vi "MultiTool-Track-Generate-ndipolarisFileOutput-Q-vectors-Accepts Joystick Command with Time Display-Testing tcp time stamp.vi"() -> ()   [LabVIEW 2013]
panel:
  out "TIME":string
  out "bytes written":i32
  out "Return time string":string
  out "Length":u8
  out "Command":u8
  out "Tool 2":T1={"Port Handle"="", "Frame Number"=0, "Tx"=0.0, "Ty"=0.0, "Tz"=0.0, "Q0"=0.0, "Qx"=0.0, "Qy"=0.0, "Qz"=0.0, "Deviation"=0.0, " Markers Missing"=TRUE, "Out of Volume"=TRUE} {"Deviation" format="%#.4f"; "Qz" format="%#.4f"; "Qy" format="%#.4f"; "Qx" format="%#.4f"; "Q0" format="%#.4f"; "Tz" format="%#.2f"; "Ty" format="%#.2f"; "Tx" format="%#.2f"}
  in  "Location of ROM File for Tool 2":path=path "C:/Program Files (x86)/Northern Digital Inc/8700339.rom"
  in  "NDI  Running":bool=TRUE
  out "Stop Reading":bool=TRUE
  out "Start Reading":bool
  out "Object Identifier":string="0"
  in  "Track Outside Measurement Volume? (F:No)":bool
  in  "Track Stray Markers? (F:No)":bool
  out "Tool 1":T1={"Port Handle"="", "Frame Number"=0, "Tx"=0.0, "Ty"=0.0, "Tz"=0.0, "Q0"=0.0, "Qx"=0.0, "Qy"=0.0, "Qz"=0.0, "Deviation"=0.0, " Markers Missing"=TRUE, "Out of Volume"=TRUE} {"Deviation" format="%#.4f"; "Qz" format="%#.4f"; "Qy" format="%#.4f"; "Qx" format="%#.4f"; "Q0" format="%#.4f"; "Tz" format="%#.2f"; "Ty" format="%#.2f"; "Tx" format="%#.2f"}
  out "TCP loop":i32
  in  "TCP Server Running":bool=TRUE
  in  "Output Directory":path=path "C:/Users/Diogo/Desktop/NDI-Labview Gripper"
  out "NDI Loop":i32
  in  "VISA resource name":refnum<visa-resource-name>="COM8"
  in  "Reset? (T:Yes)":bool=TRUE
  in  "Location of ROM File for Tool 1":path=path "C:/Program Files (x86)/Northern Digital Inc/8700449.rom"
  in  "Serial Configuration":T2={"Baud Rate (9600)"=9600, "Flow Control (0:None)"=0, "Parity"=0, "Data Bits"=8, "Stop Bits"=10} {"Stop Bits" items=["1.0"=10, "2.0"=20]; "Parity" items=["None", "Odd", "Even"]; "Flow Control (0:None)" items=["None", "XON/XOFF"]; "Baud Rate (9600)" items=["9600"=9600, "14.4k"=14400, "19.2k"=19200, "38.4k"=38400, "57.6k "=57600, "115.2k"=115200]}
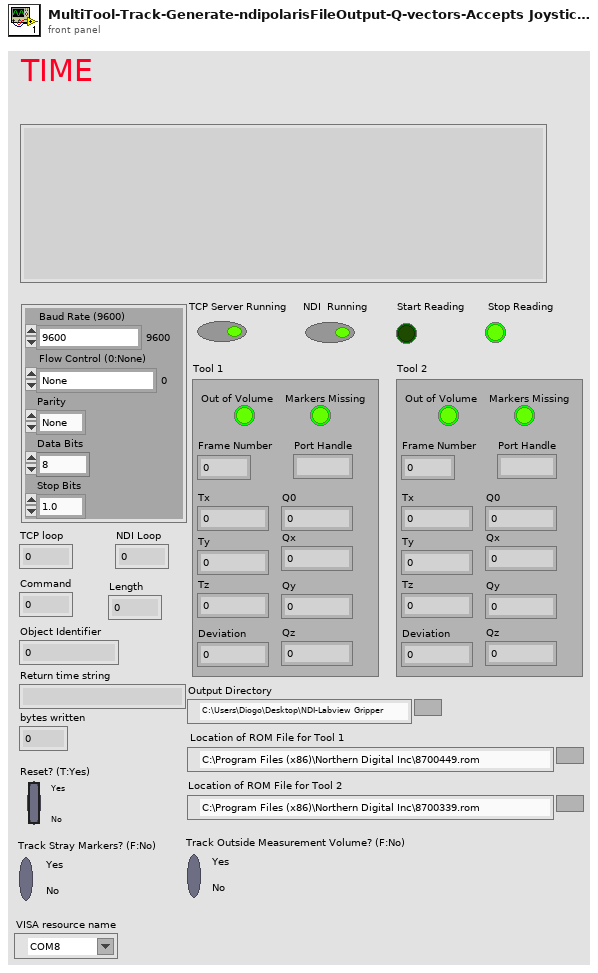
[diagram p1: front panel]
types:
  T1 = cluster{"Port Handle":string, "Frame Number":i32, "Tx":dbl, "Ty":dbl, "Tz":dbl, "Q0":dbl, "Qx":dbl, "Qy":dbl, "Qz":dbl, "Deviation":dbl, " Markers Missing":bool, "Out of Volume":bool}
  T2 = cluster{"Baud Rate (9600)":u32, "Flow Control (0:None)":u16, "Parity":u16, "Data Bits":u16, "Stop Bits":u16}
  T3 = cluster{"Port Handle":string, "Frame Number":u32, "Tx":dbl, "Ty":dbl, "Tz":dbl, "Q0":dbl, "Qx":dbl, "Qy":dbl, "Qz":dbl, "Deviation":dbl, "Missing?":bool, "Out of Volume?":bool}[]
  T4 = cluster{"Transformations[0]":cluster{"Port Handle":string, "Frame Number":u32, "Tx":dbl, "Ty":dbl, "Tz":dbl, "Q0":dbl, "Qx":dbl, "Qy":dbl, "Qz":dbl, "Deviation":dbl, "Missing?":bool, "Out of Volume?":bool}, "Transformations[1]":cluster{"Port Handle":string, "Frame Number":u32, "Tx":dbl, "Ty":dbl, "Tz":dbl, "Q0":dbl, "Qx":dbl, "Qy":dbl, "Qz":dbl, "Deviation":dbl, "Missing?":bool, "Out of Volume?":bool}, "Transformations[2]":cluster{"Port Handle":string, "Frame Number":u32, "Tx":dbl, "Ty":dbl, "Tz":dbl, "Q0":dbl, "Qx":dbl, "Qy":dbl, "Qz":dbl, "Deviation":dbl, "Missing?":bool, "Out of Volume?":bool}, "Transformations[3]":cluster{"Port Handle":string, "Frame Number":u32, "Tx":dbl, "Ty":dbl, "Tz":dbl, "Q0":dbl, "Qx":dbl, "Qy":dbl, "Qz":dbl, "Deviation":dbl, "Missing?":bool, "Out of Volume?":bool}, "Transformations[4]":cluster{"Port Handle":string, "Frame Number":u32, "Tx":dbl, "Ty":dbl, "Tz":dbl, "Q0":dbl, "Qx":dbl, "Qy":dbl, "Qz":dbl, "Deviation":dbl, "Missing?":bool, "Out of Volume?":bool}, "Transformations[5]":cluster{"Port Handle":string, "Frame Number":u32, "Tx":dbl, "Ty":dbl, "Tz":dbl, "Q0":dbl, "Qx":dbl, "Qy":dbl, "Qz":dbl, "Deviation":dbl, "Missing?":bool, "Out of Volume?":bool}, "Transformations[6]":cluster{"Port Handle":string, "Frame Number":u32, "Tx":dbl, "Ty":dbl, "Tz":dbl, "Q0":dbl, "Qx":dbl, "Qy":dbl, "Qz":dbl, "Deviation":dbl, "Missing?":bool, "Out of Volume?":bool}, "Transformations[7]":cluster{"Port Handle":string, "Frame Number":u32, "Tx":dbl, "Ty":dbl, "Tz":dbl, "Q0":dbl, "Qx":dbl, "Qy":dbl, "Qz":dbl, "Deviation":dbl, "Missing?":bool, "Out of Volume?":bool}, "Transformations[8]":cluster{"Port Handle":string, "Frame Number":u32, "Tx":dbl, "Ty":dbl, "Tz":dbl, "Q0":dbl, "Qx":dbl, "Qy":dbl, "Qz":dbl, "Deviation":dbl, "Missing?":bool, "Out of Volume?":bool}}
  T5 = cluster{"Port Handle":string, "Frame Number":u32, "Tx":dbl, "Ty":dbl, "Tz":dbl, "Q0":dbl, "Qx":dbl, "Qy":dbl, "Qz":dbl, "Deviation":dbl, "Missing?":bool, "Out of Volume?":bool}
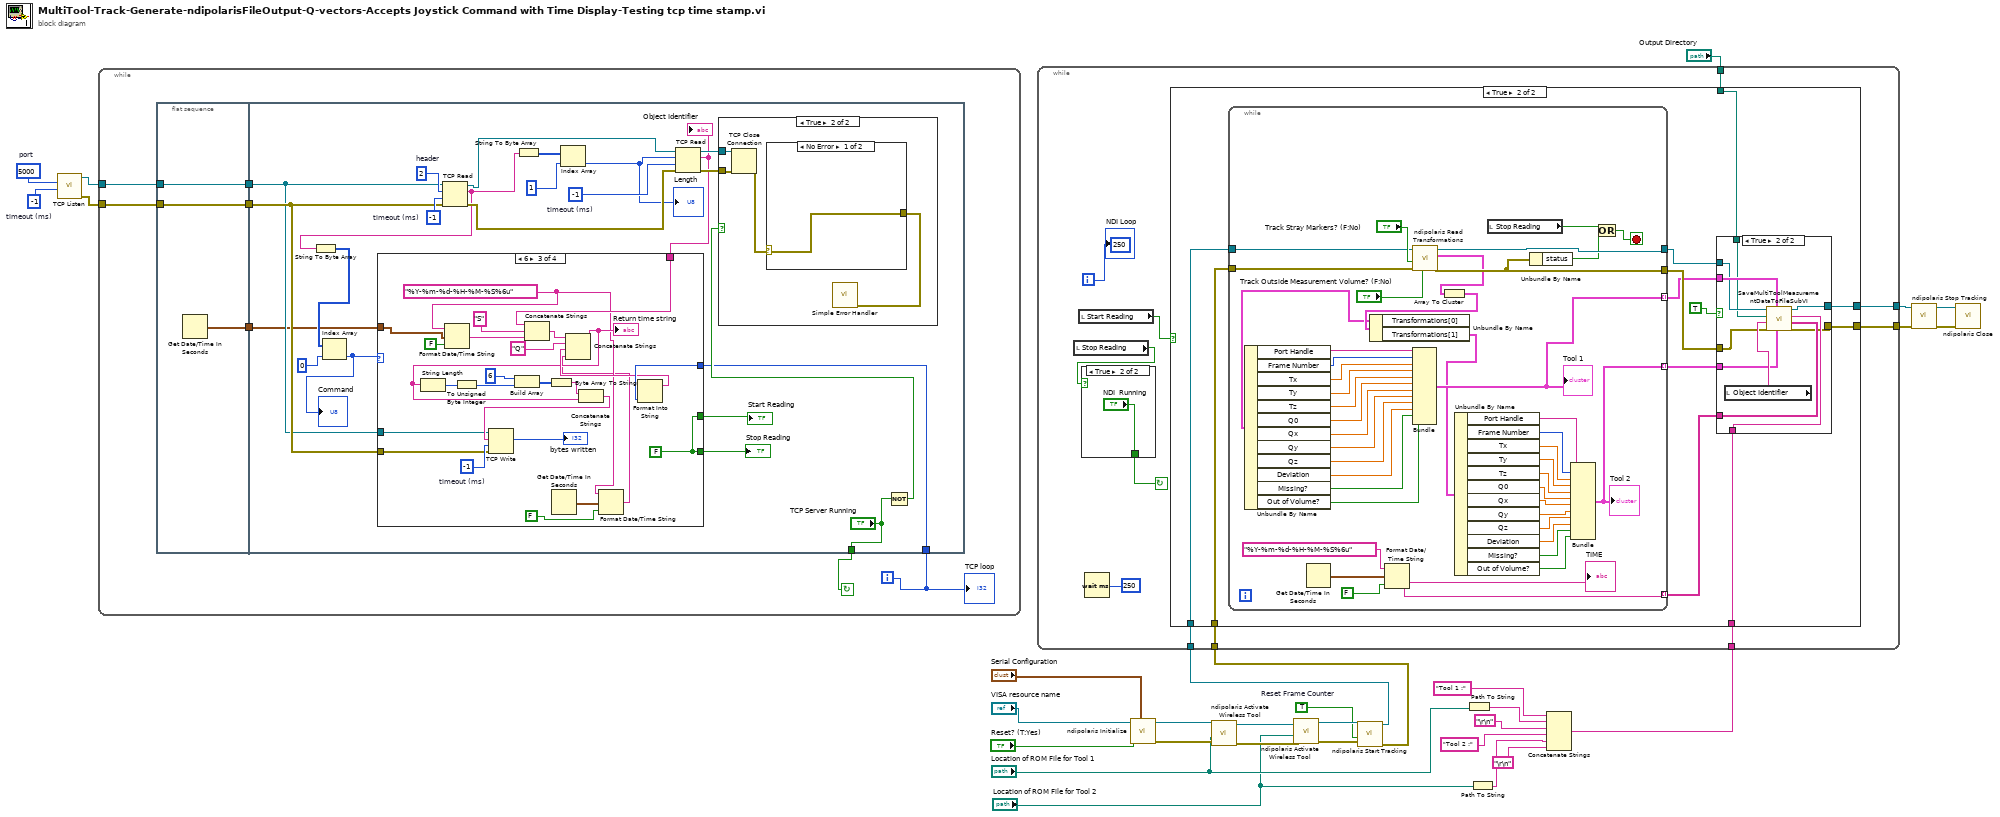
[diagram p0: block diagram]
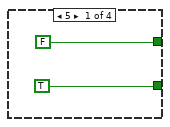
[diagram p2: hidden frame]
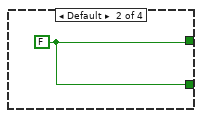
[diagram p3: hidden frame]
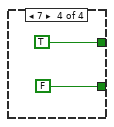
[diagram p4: hidden frame]
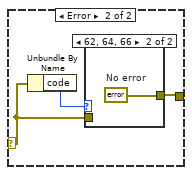
[diagram p6: hidden frame]
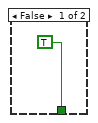
[diagram p8: hidden frame]
diagram:
  w21 = TRUE  # Reset Frame Counter
  w30 = u16 5000  # port
  w29 = i8 -1  # timeout (ms)
  n1 = call <vilib>:"TCP Listen.vi"("timeout ms (wait forever: -1)"=w29, "port"=w30) -> ("error out"=w24:errorcluster, "connection ID"=w25:refnum<k5>)  [unwired: 5 in, 3 out]
  n2 = while {
    tunnel: w25 -> [w35]
    tunnel: w24 -> [w36]
    i -> [w31]
    stop <- w37 continue-if-true
    n3 = flat-sequence {
      tunnel: w35 -> [w39]
      tunnel: w36 -> [w40]
      tunnel: [w40] -> w34
      tunnel: [w39] -> w33
      tunnel: [w38] -> w32
      tunnel: ["TCP Server Running"] -> w37
      tunnel: w34 -> [w45]
      tunnel: w33 -> [w43]
      tunnel: w32 -> [w42]
      tunnel: w31 -> [w41]
      frame #0 {
        n4 = Get Date/Time In Seconds() -> (seconds since 1Jan1904=w38:timestamp)
      }
      frame #1 {
        w59 = i8 -1  # timeout (ms)
        w62 = i8 -1  # timeout (ms)
        w63 = i8 2  # header
        n5 = TCP Read(connection ID=w43, bytes to read=w63, error in (no error)=w45, 9:w62) -> (connection ID out=w61:refnum<k5>, data out=w50:string, error out=w60:errorcluster)  [unwired: 1 in]
        n6 = String To Byte Array(string=w50) -> (unsigned byte array=w53:u8[])
        n7 = Index Array(array=w53, index=0) -> (element=w46:u8)
        "Command" <- w46
        n8 = String To Byte Array(string=w50) -> (unsigned byte array=w52:u8[])
        n9 = Index Array(array=w52, index=1) -> (element=w49:u8)
        "Length" <- w49
        n10 = TCP Read(connection ID=w61, bytes to read=w49, error in (no error)=w60, 9:w59) -> (connection ID out=w58:refnum<k5>, data out=w44:string, error out=w57:errorcluster)  [unwired: 1 in]
        "Object Identifier" <- w44
        n11 = case shown="6" w46 {
          tunnel: [FALSE w66 w77 TRUE] -> w56
          tunnel: [TRUE w66 w77 FALSE] -> w55
          tunnel: w45 -> [_ _ w80 _]
          tunnel: w44 -> [_ _ w79 _]
          tunnel: w43 -> [_ _ w78 _]
          tunnel: w42 -> [_ _ w76 _]
          tunnel: w41 -> [_ _ w73 _]
          frame 5 {
          }
          frame Default {
            w66 = FALSE
          }
          frame 6 {
            w88 = i8 -1  # timeout (ms)
            w68 = "%Y-%m-%d-%H-%M-%S%6u"
            w77 = FALSE
            n12 = Format Date/Time String(time format string (%c)=w68, seconds (now)=w76, UTC format=FALSE) -> (date/time string=w91:string)
            n13 = Concatenate Strings(w79, "S", w91) -> (w75:string)
            n14 = Get Date/Time In Seconds() -> (seconds since 1Jan1904=w70:timestamp)
            n15 = Format Date/Time String(time format string (%c)=w68, seconds (now)=w70, UTC format=FALSE) -> (date/time string=w67:string)
            n16 = Format Into String(w73) -> (resulting string=w72:string)  [unwired: 3 in, 1 out]
            n17 = Concatenate Strings(w75, "Q", w72, w67) -> (w71:string)
            "Return time string" <- w71
            n18 = String Length(string=w71) -> (length=w85:i32)
            n19 = To Unsigned Byte Integer(number=w85) -> (unsigned 8bit integer=w84:u8)
            n20 = Build Array(u8 6, w84) -> (w82:u8[])
            n21 = Byte Array To String(unsigned byte array=w82) -> (string=w87:string)
            n22 = Concatenate Strings(w87, w71) -> (w81:string)
            n23 = TCP Write(connection ID=w78, data in=w81, error in (no error)=w80, 9:w88) -> (bytes written=→"bytes written":i32)  [unwired: 2 out]
          }
          frame 7 {
          }
        }
        "Start Reading" <- w56
        "Stop Reading" <- w55
        n24 = Not(x="TCP Server Running") -> (.not. x?=w47:bool)
        n25 = case shown="True" w47 {
          tunnel: w58 -> [_ w95]
          tunnel: w57 -> [_ w94]
          frame False {
          }
          frame True {
            n26 = TCP Close Connection(connection ID=w95, error in (no error)=w94) -> (error out=w96:errorcluster)  [unwired: 1 in, 1 out]
            n27 = case shown="No Error" w96 {
              selector: w96 -> [w98 w100]
              tunnel: [w98 w99] -> w97
              frame No Error {
              }
              frame Error {
                n28 = Unbundle By Name(w100) -> ("code"=w101:i32)
                n29 = case shown="62, 64, 66" w101 {
                  tunnel: w100 -> [w102 _]
                  tunnel: [w102 w103] -> w99
                  frame Default {
                  }
                  frame 62, 64, 66 {
                    w103 = errorcluster {"status"=FALSE, "code"=0, "source"=""}  # No error
                  }
                }
              }
            }
            n30 = call <vilib>:"Simple Error Handler.vi"("error in (no error)"=w97) -> ()  [unwired: 1 in, 8 out]
          }
        }
      }
    }
    "TCP loop" <- w31
  }
  n31 = call <instrlib>:"ndipolaris Initialize.vi"("Serial Configuration"="Serial Configuration", "Reset? (T: Yes)"="Reset? (T:Yes)", "VISA resource name"="VISA resource name") -> ("error out"=w11:errorcluster, "VISA resource name out"=w12:refnum<visa-resource-name>)  [unwired: 7 in]
  n32 = call <instrlib>:"ndipolaris Activate Wireless Tool.vi"("error in (no error)"=w11, "Location of ROM File for Tool"="Location of ROM File for Tool 1", "VISA resource name"=w12) -> ("error out"=w9:errorcluster, "VISA resource out"=w10:refnum<visa-resource-name>)  [unwired: 6 in, 1 out]
  n33 = call <instrlib>:"ndipolaris Activate Wireless Tool.vi"("error in (no error)"=w9, "Location of ROM File for Tool"="Location of ROM File for Tool 2", "VISA resource name"=w10) -> ("error out"=w22:errorcluster, "VISA resource out"=w23:refnum<visa-resource-name>)  [unwired: 6 in, 1 out]
  n34 = call <instrlib>:"ndipolaris Start Tracking.vi"("error in (no error)"=w22, "Reset Frame Counter? (F:No)"=w21, "VISA resource name"=w23) -> ("error out"=w16:errorcluster, "VISA resource out"=w20:refnum<visa-resource-name>)  [unwired: 7 in]
  n35 = Path To String(path="Location of ROM File for Tool 1") -> (string=w5:string)
  n36 = Path To String(path="Location of ROM File for Tool 2") -> (string=w3:string)
  n37 = Concatenate Strings("Tool 1 :" ("string"), w5, "\r\n", "Tool 2 :" ("string"), w3, "\r\n") -> (w13:string)
  n38 = while {
    tunnel: w20 -> [w113]
    tunnel: [w112] -> w17
    tunnel: w16 -> [w111]
    tunnel: "Output Directory" -> [w110]
    tunnel: [w109] -> w14
    tunnel: w13 -> [w105]
    i -> [w114]
    stop <- w104 continue-if-true
    (unwired) u8 250
    n39 = local read "Stop Reading"() -> (w106:bool)
    n40 = local read "Start Reading"() -> (w107:bool)
    n41 = case shown="True" w106 {
      tunnel: [TRUE "NDI  Running"] -> w104
      frame False {
      }
      frame True {
      }
    }
    n42 = Wait (ms)(milliseconds to wait=u32 250) -> ()  [unwired: 1 out]
    n43 = case shown="True" w107 {
      tunnel: w113 -> [w118 w130]
      tunnel: [w118 w126] -> w112
      tunnel: w111 -> [w117 w129]
      tunnel: w110 -> [_ w128]
      tunnel: [w117 w125] -> w109
      tunnel: w105 -> [_ w120]
      frame False {
      }
      frame True {
        n44 = while {
          tunnel: [w184] -> w122
          tunnel: [w183] -> w127
          tunnel: [w160] -> w123 mode=indexing
          tunnel: [w161] -> w124 mode=indexing
          tunnel: w130 -> [w159]
          tunnel: w129 -> [w158]
          tunnel: [w143] -> w119 mode=indexing
          stop <- w185 stop-if-true
          n45 = Get Date/Time In Seconds() -> (seconds since 1Jan1904=w164:timestamp)
          n46 = Format Date/Time String(time format string (%c)="%Y-%m-%d-%H-%M-%S%6u", seconds (now)=w164, UTC format=FALSE) -> (date/time string=w161:string)
          "TIME" <- w161
          n47 = call <instrlib>:"ndipolaris Read Transformations.vi"("Track Outside Measurement Volume? (F:No)"="Track Outside Measurement Volume? (F:No)", "error in (no error)"=w158, "Track Stray Markers? (F:No)"="Track Stray Markers? (F:No)", "VISA resource name"=w159) -> ("error out"=w183:errorcluster, "Transformations"=w168:T3, "VISA resource out"=w184:refnum<visa-resource-name>)  [unwired: 4 in, 1 out]
          n48 = Array To Cluster(array=w168) -> (cluster=w179:T4)
          n49 = Unbundle By Name(w179) -> ("Transformations[0]"=w178:T5, "Transformations[1]"=w156:T5)
          n50 = Unbundle By Name(w178) -> ("Port Handle"=w177:string, "Frame Number"=w176:u32, "Tx"=w175:dbl, "Ty"=w174:dbl, "Tz"=w173:dbl, "Q0"=w172:dbl, "Qx"=w171:dbl, "Qy"=w170:dbl, "Qz"=w169:dbl, "Deviation"=w167:dbl, "Missing?"=w166:bool, "Out of Volume?"=w165:bool)
          n51 = Bundle("Port Handle"=w177, "Frame Number"=w176, "Tx"=w175, "Ty"=w174, "Tz"=w173, "Q0"=w172, "Qx"=w171, "Qy"=w170, "Qz"=w169, "Deviation"=w167, "Missing?"=w166, "Out of Volume?"=w165) -> (w160:T5)  [unwired: 1 in]
          "Tool 1" <- w160
          n52 = Unbundle By Name(w156) -> ("Port Handle"=w155:string, "Frame Number"=w154:u32, "Tx"=w153:dbl, "Ty"=w152:dbl, "Tz"=w151:dbl, "Q0"=w150:dbl, "Qx"=w149:dbl, "Qy"=w148:dbl, "Qz"=w147:dbl, "Deviation"=w146:dbl, "Missing?"=w145:bool, "Out of Volume?"=w144:bool)
          n53 = local read "Stop Reading"() -> (w157:bool)
          n54 = Unbundle By Name(w183) -> ("status"=w182:bool)
          n55 = Bundle("Port Handle"=w155, "Frame Number"=w154, "Tx"=w153, "Ty"=w152, "Tz"=w151, "Q0"=w150, "Qx"=w149, "Qy"=w148, "Qz"=w147, "Deviation"=w146, "Missing?"=w145, "Out of Volume?"=w144) -> (w143:T5)  [unwired: 1 in]
          "Tool 2" <- w143
          n56 = Or(x=w157, y=w182) -> (x .or. y?=w185:bool)
        }
        n57 = case shown="True" TRUE {
          tunnel: w128 -> [_ w140]
          tunnel: w127 -> [w131 w138]
          tunnel: [w132 w137] -> w126
          tunnel: [w131 w133] -> w125
          tunnel: w124 -> [_ w136]
          tunnel: w123 -> [_ w142]
          tunnel: w122 -> [w132 w141]
          tunnel: w120 -> [_ w135]
          tunnel: w119 -> [_ w134]
          frame False {
          }
          frame True {
            n58 = local read "Object Identifier"() -> (w139:string)
            n59 = call "SaveMultiToolMeasurementDataToFileSubVI.vi"("Array of Time for Measurement"=w136, "NDI Tool"=w135, "Array - Transformations of Tool 2"=w134, "Array - Transformations of Tool 1"=w142, "error in (no error)"=w138, "Object number"=w139, "Output Directory"=w140, "VISA Refnum in"=w141) -> ("error out"=w133:errorcluster, "VISA Refnum out"=w137:refnum<visa-resource-name>)
          }
        }
      }
    }
    "NDI Loop" <- w114
  }
  n60 = call <instrlib>:"ndipolaris Stop Tracking.vi"("error in (no error)"=w14, "VISA resource name"=w17) -> ("error out"=w18:errorcluster, "VISA resource out"=w19:refnum<visa-resource-name>)  [unwired: 8 in]
  n61 = call <instrlib>:"ndipolaris Close.vi"("error in (no error)"=w18, "VISA resource name"=w19) -> ()  [unwired: 9 in, 1 out]
